vi "Get Local Address.vi"(0 "LAN first":bool=TRUE, 9 "Excludes":string[](array[string])) -> (4 "net address":u32, 8 "address":string)   [LabVIEW 2020, in "epl-network.lvlib"]
uses:
  epl-network.lvlib
  12869db3-b163-4b27-b759-dcce922ace7e.vi
  e71cd835-4f44-4a9b-b5db-a75600b7108d.vi
  <vilib>/Comparison/Equal/Equal Functor/Equal Functor.lvclass
  <vilib>/Comparison/Less/Less Functor/Less Functor.lvclass
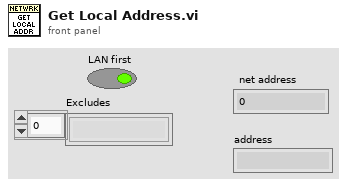
[diagram p1: front panel]
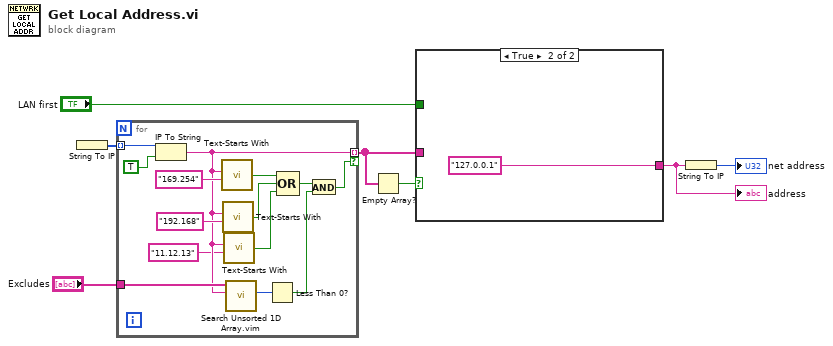
[diagram p0: block diagram]
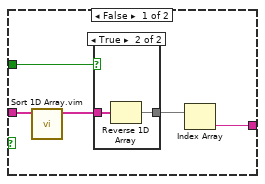
[diagram p2: hidden frame]
diagram:
  n1 = String To IP() -> (0:w4:u32[])  [unwired: 1 in]
  n2 = for {
    tunnel: w4 -> [w20] mode=indexing
    tunnel: [w10] -> w6 mode=indexing if=w13
    tunnel: "Excludes" -> [w14]
    n3 = IP To String(1:TRUE ("dot notation? (F)"), 2:w20) -> (0:w10:string)
    n4 = call "Text-Starts With.vi"("Starts with"="169.254", "String"=w10) -> ("result"=w17:bool)  [unwired: 4 in]
    n5 = call "Text-Starts With.vi"("Starts with"="192.168", "String"=w10) -> ("result"=w15:bool)  [unwired: 4 in]
    n6 = call "Text-Starts With.vi"("Starts with"="11.12.13", "String"=w10) -> ("result"=w8:bool)  [unwired: 4 in]
    n7 = call "Search Unsorted 1D Array.vim"("element"=w10, "unsorted 1D array"=w14) -> ("index of element"=w12:i32)  [unwired: 9 in]
    n8 = Less Than 0?(x=w12) -> (x < 0?=w11:bool)
    n9 = Compound Arithmetic op=OR(w17, w15, w8) -> (w16:bool)
    n10 = And(x=w16, y=w11) -> (x .and. y?=w13:bool)
  }
  n11 = Empty Array?(array=w6) -> (empty?=w7:bool)
  n12 = case shown="True" w7 {
    tunnel: w6 -> [w25 _]
    tunnel: [w26 "127.0.0.1"] -> w1
    tunnel: "LAN first" -> [w22 _]
    frame False {
      n13 = call "Sort 1D Array.vim"("unsorted array"=w25) -> ("sorted array"=w24:string[])  [unwired: 10 in]
      n14 = case shown="True" w22 {
        tunnel: w24 -> [w27 w29]
        tunnel: [w27 w28] -> w23
        frame False {
        }
        frame True {
          n15 = Reverse 1D Array(array=w29) -> (reversed array=w28:string[])
        }
      }
      n16 = Index Array(array=w23) -> (element=w26:string)  [unwired: 1 in]
    }
    frame True {
    }
  }
  "address" <- w1
  n17 = String To IP(1:w1) -> (0:→"net address":u32)
